vi "Properties.vi"() -> ()   [LabVIEW 2015, in "Engine Simulation Toolkit Shared.lvlib"]
doc: "Use this Global VI to access the GUIDs assigned to the page resources of the Custom Device."
uses:
  Engine Simulation Toolkit Shared.lvlib
panel:
  in  "Tab Control":T1(tab)=enum."Dir Speed"
  in  "Main.Master RIO Device":string="Main.Master RIO Device"
  in  "Main.Bitfiles":string="Main.Bitfiles"
  in  "Main.DirSpeed Sensor":string="Main.DirSpeed Sensor"
  in  "Main.APUs":string="Main.APUs"
  in  "Main.Knock Sensor":string="Main.Knock Sensor"
  in  "Main.Knock Cylinder":string="Main.Knock Cylinder"
  in  "Main.CompiledData":string="Main.CompiledData"
  in  "Main.CPU":string="Main.CPU"
  in  "Main.validBitfile":string="Main.validBitfile"
  in  "IP.bitfile name":string="IP.bitfile name"
  in  "Main.bitfile EPS version":string="Main.bitfile EPS version"
  in  "Main.ETiming Meas":string="Main.ETiming Meas"
  in  "Main.Digital PatGens":string="Main.Digital PatGens"
  in  "Main.ETiming Caps":string="Main.ETiming Caps"
  in  "Main.Analog Replays":string="Main.Analog Replays"
  in  "Main.Bitfile":string="Main.Bitfile"
  in  "Main.Device Address":string="Main.Device Address"
  in  "Engine.accel on":string="Engine.accel on"
  in  "Engine.accel val":string="Engine.accel val"
  in  "Engine.start angle":string="Engine.start angle"
  in  "Engine.rotations":string="Engine.rotations"
  in  "DataReplay.VBelowMin":string="DataReplay.VBelowMin"
  in  "DataReplay.DACRange":string="DataReplay.DACRange"
  in  "DataReplay.VOverride":string="DataReplay.VOverride"
  in  "DataReplay.ReverseNegate":string="DataReplay.ReverseNegate"
  in  "DataReplay.Reverse":string="DataReplay.Reverse"
  in  "DataReplay.FileLength":string="DataReplay.FileLength"
  in  "DataReplay.FileOffset":string="DataReplay.FileOffset"
  in  "DataReplay.FileMethod":string="DataReplay.FileMethod"
  in  "DataReplay.FileDataPlugin":string="DataReplay.FileDataPlugin"
  in  "DataReplay.FileChannel":string="DataReplay.FileChannel"
  in  "DataReplay.FileGroup":string="DataReplay.FileGroup"
  in  "DataReplay.File":string="DataReplay.File"
  in  "DataReplay.MissingLocation":string="DataReplay.MissingLocation"
  in  "DataReplay.VatMin":string="DataReplay.VatMin"
  in  "DataReplay.VatMax":string="DataReplay.VatMax"
  in  "DataReplay.PositionRef":string="DataReplay.PositionRef"
  in  "DataReplay.MaxSpeed":string="DataReplay.MaxSpeed"
  in  "DataReplay.MinSpeed":string="DataReplay.MinSpeed"
  in  "DataReplay.MemSize":string="DataReplay.MemSize"
  in  "ETiming.RefSelect":string="ETiming.RefSelect"
  in  "ETiming.WindowRefs":string="ETiming.WindowRefs"
  in  "ETiming.DefaultEnd":string="ETiming.DefaultEnd"
  in  "ETiming.DefaultStart":string="ETiming.DefaultStart"
  in  "ETiming.ReferenceAngle":string="ETiming.ReferenceAngle"
  in  "ETiming.MeasActiveLimit":string="ETiming.MeasActiveLimit"
  in  "ETiming.MeasPolarity":string="ETiming.MeasPolarity"
  in  "ETiming.MeasWindowName":string="ETiming.MeasWindowName"
  in  "ETiming.WindowMaxs":string="ETiming.WindowMaxs"
  in  "ETiming.WindowMins":string="ETiming.WindowMins"
  in  "ETiming.WindowNames":string="ETiming.WindowNames"
  in  "DigPattrn.Add_Width_":string="DigPattrn.Add_Width_"
  in  "DigPattrn.Add_Offset_":string="DigPattrn.Add_Offset_"
  in  "DigPattrn.Add_Tooth_":string="DigPattrn.Add_Tooth_"
  in  "DigPattrn.Rem_Edge_":string="DigPattrn.Rem_Edge_"
  in  "DigPattrn.Rem_Tooth_":string="DigPattrn.Rem_Tooth_"
  in  "DigPattrn.Offset":string="DigPattrn.Offset"
  in  "DigPattrn.Width":string="DigPattrn.Width"
  in  "DigPattrn.Teeth":string="DigPattrn.Teeth"
  in  "DigPattrn.Length":string="DigPattrn.Length"
  in  "Knock.MaxSpeed":string="Knock.MaxSpeed"
  in  "Knock.MinFreq":string="Knock.MinFreq"
  in  "Knock.MaxFreq":string="Knock.MaxFreq"
  in  "Knock.LowFreqMode":string="Knock.LowFreqMode"
  in  "Knock.HighFreq":string="Knock.HighFreq"
  in  "Knock.DACRange":string="Knock.DACRange"
  in  "Knock.Duration":string="Knock.Duration"
  in  "Knock.LowFreq":string="Knock.LowFreq"
  in  "DirSpeed.ToothSource":string="DirSpeed.ToothSource"
  # "Use `Get Bitfile Property Name.vi`\nto get the property name for\na specific bitfile path; it is derived\nfrom Main.Bitfiles."
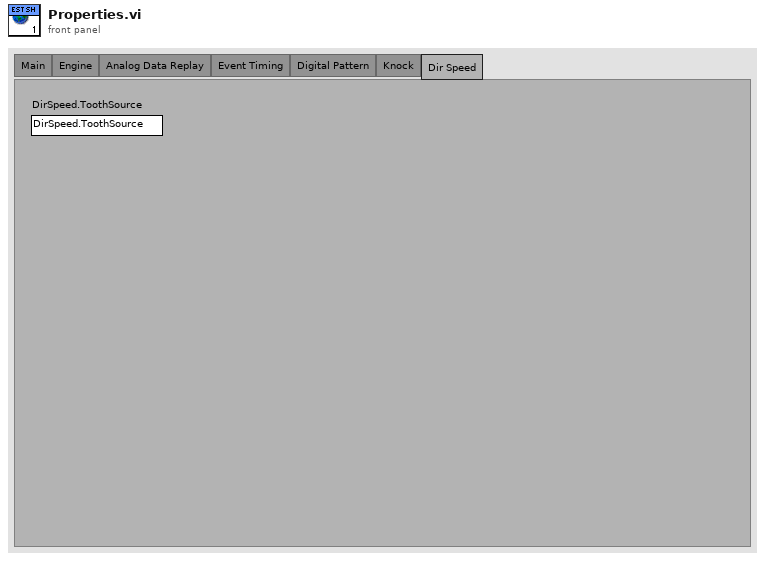
[diagram p1: front panel]
types:
  T1 = enum32{"Main", "Engine", "Analog Data Replay", "Event Timing", "Digital Pattern", "Knock", "Dir Speed"}
diagram:
